vi "例程33-仿真信号ExpressVI的使用.vi"() -> ()   [LabVIEW 2016]
panel:
  out "error out 2":errorcluster caption="错误输出"
  out "正弦与均匀噪声 2":dynamicdata(graph) caption="正弦与均匀噪声"
  in  "Seed Number 2":dbl=-1.0 caption="种子值"
  in  "噪声幅值 2":dbl=0.6 caption="噪声幅值"
  in  "error in (no error) 2":errorcluster caption="错误输入（无错误）"
  in  "Phase 2":dbl caption="相位"
  in  "Amplitude 2":dbl=1.0 caption="幅值"
  in  "Frequency 2":dbl=10.1 caption="频率"
  in  "Reset Signal 2":bool caption="重置信号"
  in  "Offset 2":dbl caption="偏移量"
  out "error out":errorcluster caption="错误输出"
  out "正弦与均匀噪声":dynamicdata(graph)
  in  "Seed Number":dbl=-1.0 caption="种子值"
  in  "噪声幅值":dbl=0.6
  in  "error in (no error)":errorcluster caption="错误输入（无错误）"
  in  "Phase":dbl caption="相位"
  in  "Amplitude":dbl=1.0 caption="幅值"
  in  "Frequency":dbl=10.1 caption="频率"
  in  "Reset Signal":bool caption="重置信号"
  in  "Offset":dbl caption="偏移量"
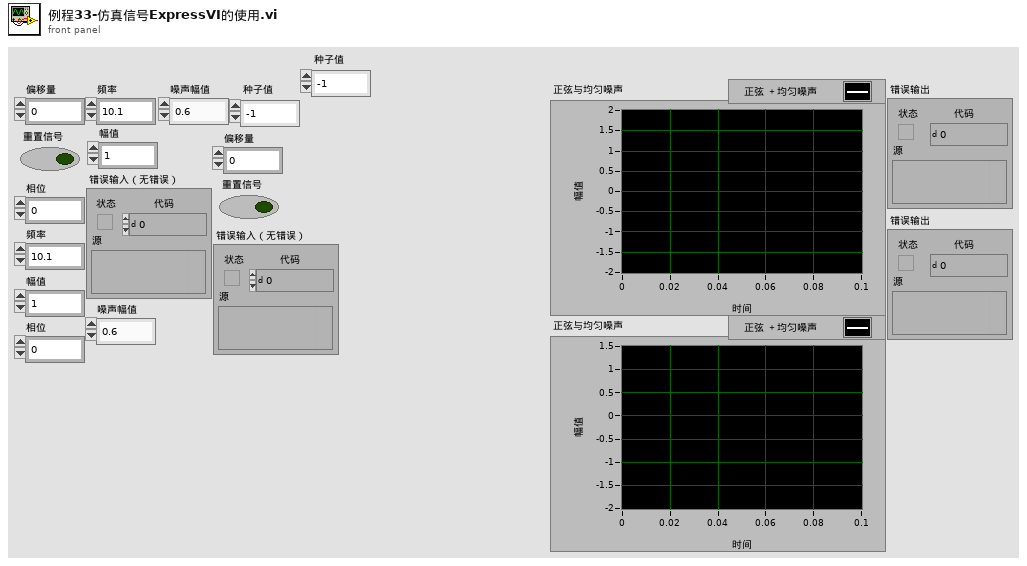
[diagram p1: front panel]
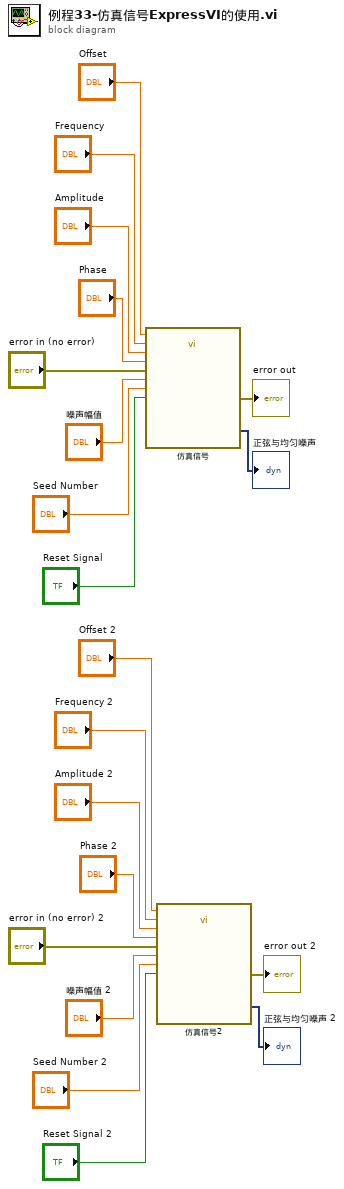
[diagram p0: block diagram]
diagram:
  n1 = call "仿真信号"("Offset"="Offset", "Reset Signal"="Reset Signal", "Frequency"="Frequency", "Amplitude"="Amplitude", "Phase"="Phase", "error in (no error)"="error in (no error)", "噪声幅值"="噪声幅值", "Seed Number"="Seed Number") -> ("正弦与均匀噪声"=→"正弦与均匀噪声":dynamicdata, "error out"=→"error out":errorcluster)  [unwired: 6 in]
  n2 = call "仿真信号2"("Offset"="Offset 2", "Reset Signal"="Reset Signal 2", "Frequency"="Frequency 2", "Amplitude"="Amplitude 2", "Phase"="Phase 2", "error in (no error)"="error in (no error) 2", "噪声幅值"="噪声幅值 2", "Seed Number"="Seed Number 2") -> ("正弦与均匀噪声"=→"正弦与均匀噪声 2":dynamicdata, "error out"=→"error out 2":errorcluster)  [unwired: 6 in]
